vi "Detector Status.vi"(7 "Address":u16, 8 "Error In":errorcluster, 10 "Detector":u8, 11 "VISA Resource in":refnum<visa-resource-name>) -> (0 "Error Out":errorcluster, 1 "Detector Cluster":T1, 2 "Detector Status":u8 format="%.0b", 3 "VISA Resource out":refnum<visa-resource-name>)   [LabVIEW 2014, in "KIT QV.lvlib"]
doc: "Status of selected detector."
uses:
  KIT QV.lvlib
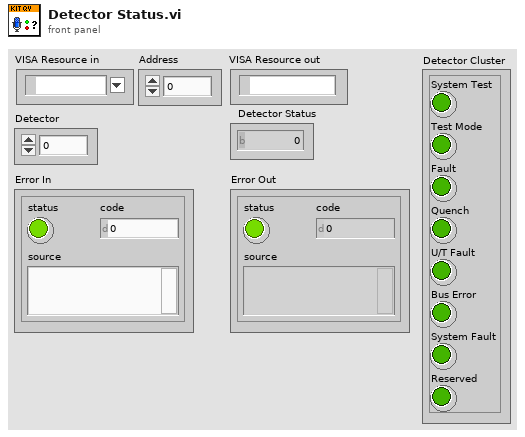
[diagram p1: front panel]
types:
  T1 = cluster{"System Test":bool, "Test Mode":bool, "Fault":bool, "Quench":bool, "U/T Fault":bool, "Bus Error":bool, "System Fault":bool, "Reserved":bool}
  T2 = cluster{"[0]":bool, "[1]":bool, "[2]":bool, "[3]":bool, "[4]":bool, "[5]":bool, "[6]":bool, "[7]":bool}
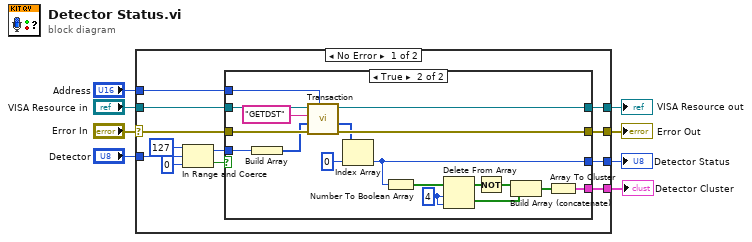
[diagram p0: block diagram]
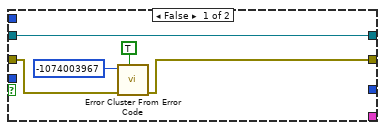
[diagram p2: hidden frame]
diagram:
  n1 = case shown="No Error" "Error In" {
    selector: "Error In" -> [w19 w44]
    tunnel: [w17 w45] -> w8
    tunnel: [w16 w44] -> w7
    tunnel: "VISA Resource in" -> [w20 w45]
    tunnel: "Address" -> [w18 _]
    tunnel: [w15 _] -> w3
    tunnel: [w14 _] -> w2
    tunnel: "Detector" -> [w11 _]
    frame No Error {
      n2 = In Range and Coerce(upper limit=u8 127, x=w11, lower limit=u8 0) -> (coerced(x)=w9:u8, In Range?=w10:bool)
      n3 = case shown="True" w10 {
        tunnel: w20 -> [w25 w43]
        tunnel: w19 -> [w22 w42]
        tunnel: w18 -> [_ w40]
        tunnel: [w25 w39] -> w17
        tunnel: [w21 w38] -> w16
        tunnel: [_ w35] -> w15
        tunnel: [_ w26] -> w14
        tunnel: w9 -> [_ w34]
        frame False {
          n4 = call <vilib>:"Error Cluster From Error Code.vi"("show call chain? (False)"=TRUE, "error in (no error)"=w22, "error code (0)"=-1074003967) -> ("error out"=w21:errorcluster)  [unwired: 6 in]
        }
        frame True {
          w31 = 4 ("length")
          n5 = Build Array(w34) -> (w33:u8[])
          n6 = call "Transaction.vi"("Address"=w40, "error in (no error)"=w42, "Parameter in"=w33, "Command"="GETDST" ("Reset Command"), "VISA Resource in"=w43) -> ("error out"=w38:errorcluster, "Parameter out"=w37:u8[], "VISA Resource out"=w39:refnum<visa-resource-name>)  [unwired: 4 in]
          n7 = Index Array(array=w37, index=0) -> (element=w35:u8)
          n8 = Number To Boolean Array(number=w35) -> (Boolean array=w32:bool[])
          n9 = Delete From Array(array=w32, length=w31, index=w31) -> (deleted portion=w27:bool[], array with subset deleted=w30:bool[])
          n10 = Not(x=w30) -> (.not. x?=w28:bool[])
          n11 = Build Array (concatenate)(w28, w27) -> (w29:bool[])
          n12 = Array To Cluster(array=w29) -> (cluster=w26:T2)
        }
      }
    }
    frame Error {
    }
  }
  "Error Out" <- w7
  "VISA Resource out" <- w8
  "Detector Status" <- w3
  "Detector Cluster" <- w2
